vi "NPMManager.vi"(3 "error in (no error)":errorcluster caption="错误输入（无错误）", 4 "Input":T2, 5 "ref_in":T1) -> (0 "error out":errorcluster caption="错误输出", 1 "Output":T2, 2 "ref_out":T1)   [LabVIEW 2012]
uses:
  D:/workspace/GitHub/LVsolis/lib/CmdLib.dll
  lib/CmdLib.dll
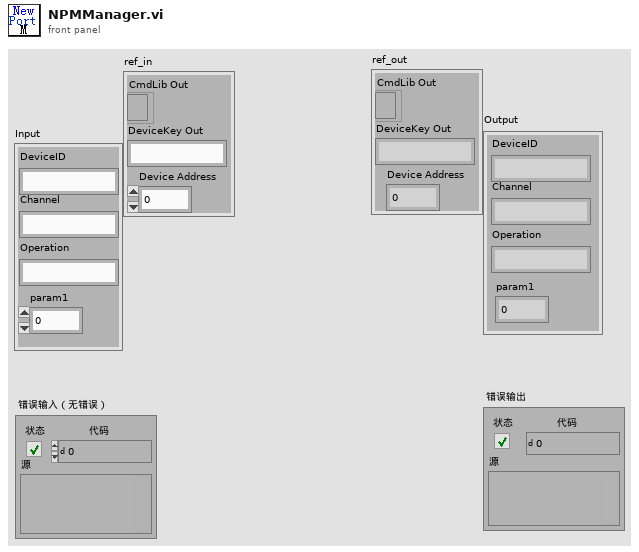
[diagram p1: front panel]
types:
  T1 = cluster{"CmdLib Out":refnum<k24>, "DeviceKey Out":string, "Device Address":i32}
  T2 = cluster{"DeviceID":string, "Channel":string, "param1":dbl, "Operation":string}
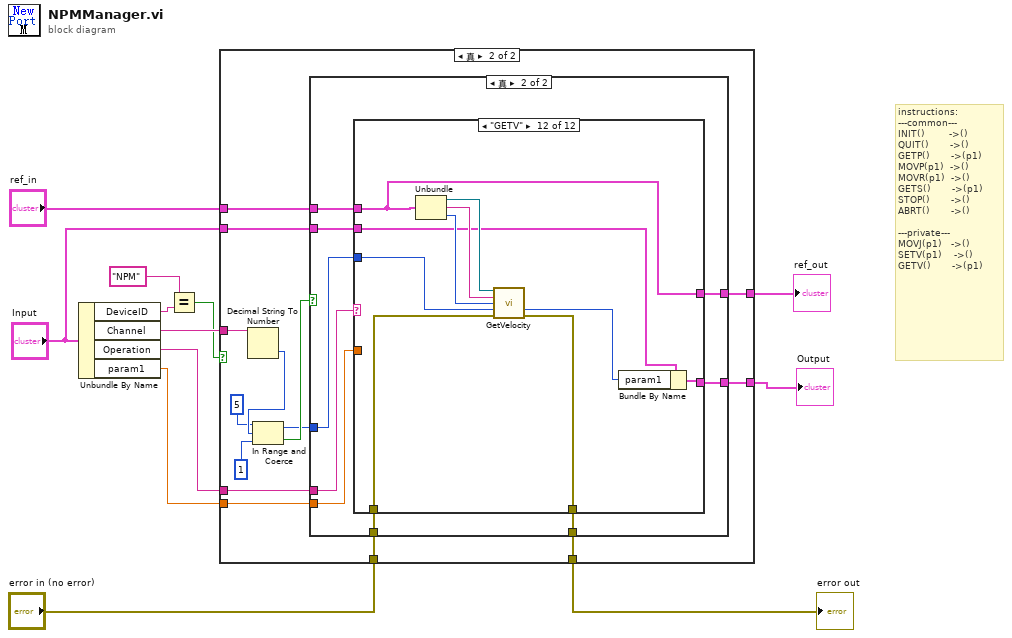
[diagram p0: block diagram]
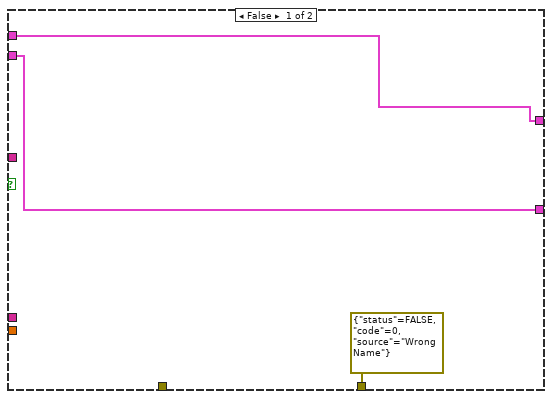
[diagram p2: hidden frame]
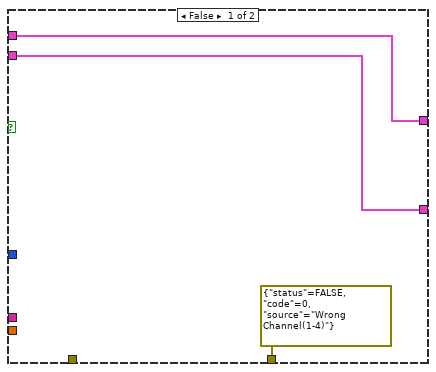
[diagram p3: hidden frame]
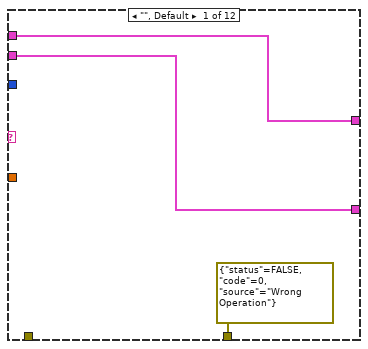
[diagram p4: hidden frame]
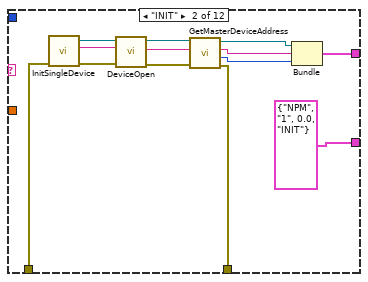
[diagram p5: hidden frame]
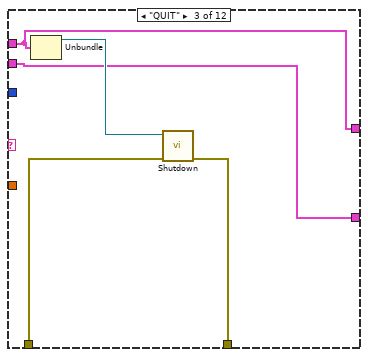
[diagram p6: hidden frame]
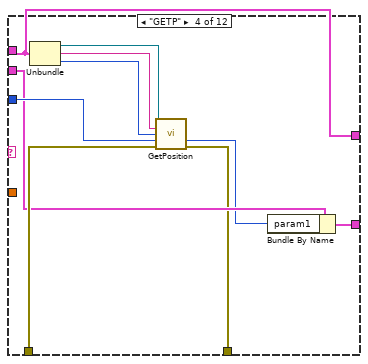
[diagram p7: hidden frame]
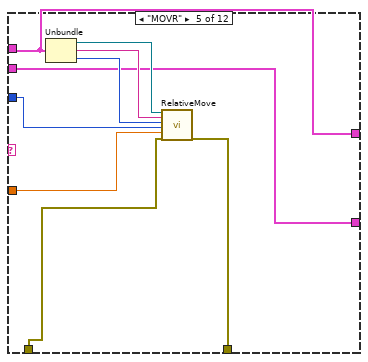
[diagram p8: hidden frame]
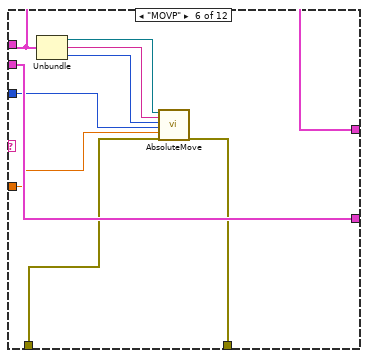
[diagram p9: hidden frame]
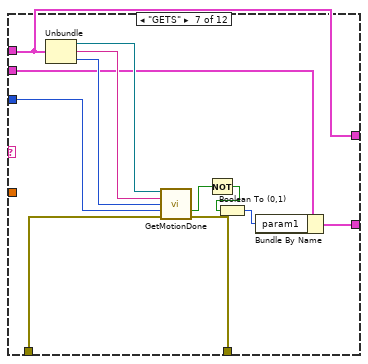
[diagram p10: hidden frame]
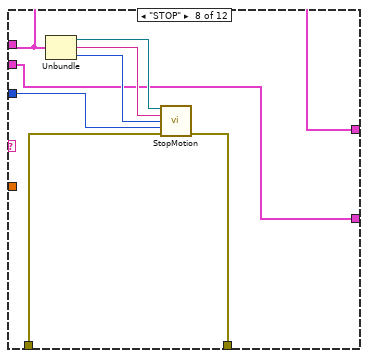
[diagram p11: hidden frame]
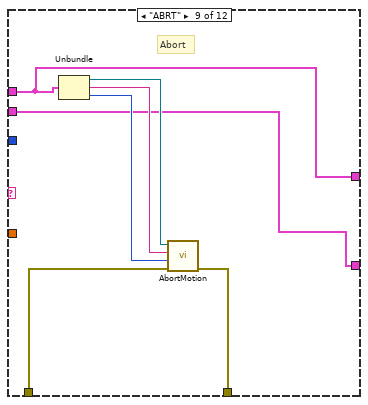
[diagram p12: hidden frame]
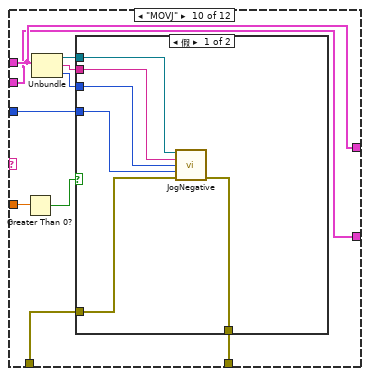
[diagram p13: hidden frame]
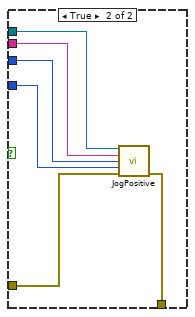
[diagram p14: hidden frame]
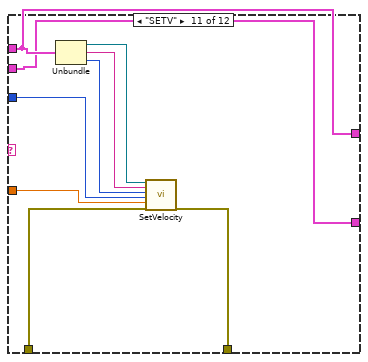
[diagram p15: hidden frame]
diagram:
  # "instructions:\n---common---\nINIT()        ->()\nQUIT()       ->()\nGETP()       ->(p1)\nMOVP(p1)  ->()\nMOVR(p1)  ->()\nGETS()       ->(p1)\nSTOP()       ->()\nABRT()       ->()\n\n---private---\nMOVJ(p1)   ->()\nSETV(p1)    ->()\nGETV()       ->(p1)"
  n1 = Unbundle By Name("Input") -> ("DeviceID"=w12:string, "Channel"=w10:string, "Operation"=w9:string, "param1"=w8:dbl)
  n2 = Equal?(x="NPM", y=w12) -> (x = y?=w1:bool)
  n3 = case shown="真" w1 {
    tunnel: w10 -> [_ w29]
    tunnel: w9 -> [_ w23]
    tunnel: w8 -> [_ w22]
    tunnel: [w15 w21] -> w7
    tunnel: "error in (no error)" -> [_ w20]
    tunnel: [errorcluster {"status"=FALSE, "code"=0, "source"="Wrong Name"} ("error out") w19] -> w5
    tunnel: [w14 w18] -> w4
    tunnel: "ref_in" -> [w15 w17]
    tunnel: "Input" -> [w14 w16]
    frame False {
    }
    frame True {
      n4 = Decimal String To Number(string=w29) -> (number=w28:i32)  [unwired: 2 in, 1 out]
      n5 = In Range and Coerce(upper limit=5 ("上限"), x=w28, lower limit=1 ("下限")) -> (coerced(x)=w24:i32, In Range?=w25:bool)
      n6 = case shown="真" w25 {
        tunnel: w24 -> [_ w40]
        tunnel: w23 -> [_ w41]
        tunnel: w22 -> [_ w39]
        tunnel: [w32 w38] -> w21
        tunnel: w20 -> [_ w37]
        tunnel: [errorcluster {"status"=FALSE, "code"=0, "source"="Wrong Channel(1-4)"} ("error out") w36] -> w19
        tunnel: [w31 w35] -> w18
        tunnel: w17 -> [w32 w34]
        tunnel: w16 -> [w31 w33]
        frame False {
        }
        frame True {
          n7 = case shown="\"GETV\"" w41 {
            tunnel: w40 -> [_ _ _ w69 w80 w86 w99 w107 _ w122 w145 w155]
            tunnel: w39 -> [_ _ _ _ w81 w85 _ _ _ w127 w144 _]
            tunnel: [w44 w48 w59 w67 w73 w84 w96 w104 w111 w119 w141 w152] -> w38
            tunnel: w37 -> [_ w47 w61 w68 w76 w83 w98 w106 w114 w121 w143 w154]
            tunnel: [errorcluster {"status"=FALSE, "code"=0, "source"="Wrong Operation"} ("error out") w46 w60 w63 w75 w82 w97 w105 w113 w120 w142 w153] -> w36
            tunnel: [w43 T2 {"DeviceID"="NPM", "Channel"="1", "param1"=0.0, "Operation"="INIT"} ("Output") w58 w64 w74 w90 w94 w103 w112 w118 w140 w149] -> w35
            tunnel: w34 -> [w44 _ w59 w67 w73 w84 w96 w104 w111 w119 w141 w152]
            tunnel: w33 -> [w43 _ w58 w66 w74 w90 w95 w103 w112 w118 w140 w151]
            frame "", Default {
            }
            frame "INIT" {
              n8 = call "InitSingleDevice.vi"("error in (no error)"=w47) -> ("error out"=w57:errorcluster, "DeviceKey Out"=w52:string, "CmdLib Out"=w53:refnum<k24>)  [unwired: 4 in]
              n9 = call "DeviceOpen.vi"("error in (no error)"=w57, "DeviceKey In"=w52, "CmdLib In"=w53) -> ("error out"=w56:errorcluster, "DeviceKey Out"=w55:string, "CmdLib Out"=w54:refnum<k24>)  [unwired: 2 in]
              n10 = call "GetMasterDeviceAddress.vi"("error in (no error)"=w56, "DeviceKey In"=w55, "CmdLib In"=w54) -> ("error out"=w46:errorcluster, "Device Address"=w49:i32, "DeviceKey Out"=w50:string, "CmdLib Out"=w51:refnum<k24>)  [unwired: 1 in]
              n11 = Bundle("CmdLib Out"=w51, "DeviceKey Out"=w50, "Device Address"=w49) -> (w48:T1)  [unwired: 1 in]
            }
            frame "QUIT" {
              n12 = Unbundle(w59) -> ("CmdLib Out"=w62:refnum<k24>)  [unwired: 2 out]
              n13 = call "Shutdown.vi"("error in (no error)"=w61, "CmdLib In"=w62) -> ("error out"=w60:errorcluster)  [unwired: 4 in, 1 out]
            }
            frame "GETP" {
              n14 = Unbundle(w67) -> ("CmdLib Out"=w72:refnum<k24>, "DeviceKey Out"=w71:string, "Device Address"=w70:i32)
              n15 = call "GetPosition.vi"("CmdLib In"=w72, "DeviceKey In"=w71, "Device Address In"=w70, "Motor"=w69, "error in (no error)"=w68) -> ("Position"=w65:i32, "error out"=w63:errorcluster)  [unwired: 6 in, 3 out]
              n16 = Bundle By Name(cluster=w66, "param1"=w65) -> (w64:T2)
            }
            frame "MOVR" {
              n17 = Unbundle(w73) -> ("CmdLib Out"=w79:refnum<k24>, "DeviceKey Out"=w78:string, "Device Address"=w77:i32)
              n18 = call "RelativeMove.vi"("CmdLib In"=w79, "DeviceKey In"=w78, "Device Address In"=w77, "Motor"=w80, "Relative Steps"=w81, "error in (no error)"=w76) -> ("error out"=w75:errorcluster)  [unwired: 10 in, 3 out]
            }
            frame "MOVP" {
              n19 = Unbundle(w84) -> ("CmdLib Out"=w89:refnum<k24>, "DeviceKey Out"=w88:string, "Device Address"=w87:i32)
              n20 = call "AbsoluteMove.vi"("CmdLib In"=w89, "DeviceKey In"=w88, "Device Address In"=w87, "Motor"=w86, "Target Pos"=w85, "error in (no error)"=w83) -> ("error out"=w82:errorcluster)  [unwired: 10 in, 3 out]
            }
            frame "GETS" {
              n21 = Unbundle(w96) -> ("CmdLib Out"=w102:refnum<k24>, "DeviceKey Out"=w101:string, "Device Address"=w100:i32)
              n22 = call "GetMotionDone.vi"("CmdLib In"=w102, "DeviceKey In"=w101, "Device Address In"=w100, "Motor"=w99, "error in (no error)"=w98) -> ("Is Motion Done"=w92:bool, "error out"=w97:errorcluster)  [unwired: 6 in, 3 out]
              n23 = Not(x=w92) -> (.not. x?=w91:bool)
              n24 = Boolean To (0,1)(Boolean=w91) -> (0, 1=w93:i16)
              n25 = Bundle By Name(cluster=w95, "param1"=w93) -> (w94:T2)
            }
            frame "STOP" {
              n26 = Unbundle(w104) -> ("CmdLib Out"=w110:refnum<k24>, "DeviceKey Out"=w109:string, "Device Address"=w108:i32)
              n27 = call "StopMotion.vi"("CmdLib In"=w110, "DeviceKey In"=w109, "Device Address In"=w108, "Motor"=w107, "error in (no error)"=w106) -> ("error out"=w105:errorcluster)  [unwired: 7 in, 3 out]
            }
            frame "ABRT" {
              # "Abort"
              n28 = Unbundle(w111) -> ("CmdLib Out"=w117:refnum<k24>, "DeviceKey Out"=w116:string, "Device Address"=w115:i32)
              n29 = call "AbortMotion.vi"("error in (no error)"=w114, "Device Address In"=w115, "DeviceKey In"=w116, "CmdLib In"=w117) -> ("error out"=w113:errorcluster)  [unwired: 3 out]
            }
            frame "MOVJ" {
              n30 = Greater Than 0?(x=w127) -> (x > 0?=w126:bool)
              n31 = Unbundle(w119) -> ("CmdLib Out"=w125:refnum<k24>, "DeviceKey Out"=w124:string, "Device Address"=w123:i32)
              n32 = case shown="假" w126 {
                tunnel: w125 -> [w133 w139]
                tunnel: w124 -> [w132 w138]
                tunnel: w123 -> [w131 w137]
                tunnel: w122 -> [w130 w136]
                tunnel: w121 -> [w129 w135]
                tunnel: [w128 w134] -> w120
                frame False {
                  n33 = call "JogNegative.vi"("CmdLib In"=w133, "DeviceKey In"=w132, "Device Address In"=w131, "Motor"=w130, "error in (no error)"=w129) -> ("error out"=w128:errorcluster)  [unwired: 7 in, 3 out]
                }
                frame True {
                  n34 = call "JogPositive.vi"("CmdLib In"=w139, "DeviceKey In"=w138, "Device Address In"=w137, "Motor"=w136, "error in (no error)"=w135) -> ("error out"=w134:errorcluster)  [unwired: 7 in, 3 out]
                }
              }
            }
            frame "SETV" {
              n35 = Unbundle(w141) -> ("CmdLib Out"=w148:refnum<k24>, "DeviceKey Out"=w147:string, "Device Address"=w146:i32)
              n36 = call "SetVelocity.vi"("CmdLib In"=w148, "DeviceKey In"=w147, "Device Address In"=w146, "Motor"=w145, "Steps Per Sec"=w144, "error in (no error)"=w143) -> ("error out"=w142:errorcluster)  [unwired: 10 in, 3 out]
            }
            frame "GETV" {
              n37 = Unbundle(w152) -> ("CmdLib Out"=w158:refnum<k24>, "DeviceKey Out"=w157:string, "Device Address"=w156:i32)
              n38 = call "GetVelocity.vi"("CmdLib In"=w158, "DeviceKey In"=w157, "Device Address In"=w156, "Motor"=w155, "error in (no error)"=w154) -> ("Steps Per Sec"=w150:i32, "error out"=w153:errorcluster)  [unwired: 6 in, 3 out]
              n39 = Bundle By Name(cluster=w151, "param1"=w150) -> (w149:T2)
            }
          }
        }
      }
    }
  }
  "Output" <- w4
  "error out" <- w5
  "ref_out" <- w7
